vi "readLogStatusChecks.vi"(8 "error in (no error)":errorcluster, 10 "Parser":refnum<class "U8ArrayParserAutoIndexing.lvclass">, 11 "M1M3SAL in":refnum<class "M1M3SAL.lvclass">) -> (0 "error out":errorcluster, 2 "EventStatusChecks":variant, 3 "M1M3SAL out":refnum<class "M1M3SAL.lvclass">)   [LabVIEW 2016, in "M1M3SupportCommunicator.lvlib" / "M1M3SAL.lvclass"]
uses:
  M1M3SAL.lvclass
  Common_RT_Utilities/U8ArrayParserAutoIndexing/U8ArrayParserAutoIndexing.lvclass
  DataTypes/Topics/EventStatusChecks.ctl
  DataTypes/Topics/Parts/Timestamp.ctl
  DataTypes/Topics/M1M3SupportTopics.lvlib
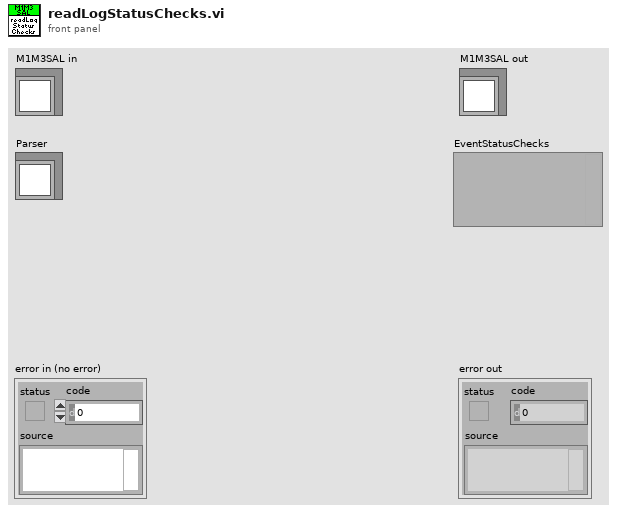
[diagram p1: front panel]
types:
  T1 = typedef "M1M3SupportTopics.lvlib/EventStatusChecks.ctl" = cluster{"Timestamp":T2, "ILCResetOk":bool, "DCAResetOk":bool, "ILCPowerOk":bool, "DCAPowerOk":bool}
  T2 = typedef "M1M3SupportTopics.lvlib/Timestamp.ctl" = dbl
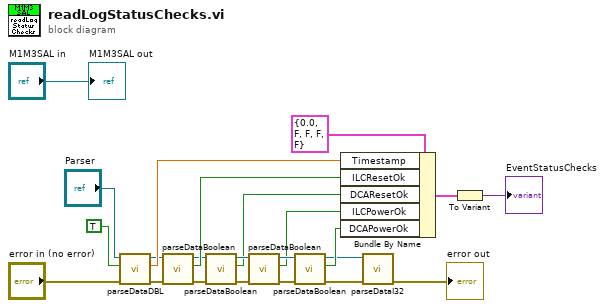
[diagram p0: block diagram]
diagram:
  n1 = call "parseDataDBL.vi"("error in (no error)"="error in (no error)", "OverrideSwapBytes"=TRUE, "U8ArrayParserAutoIndexing in"="Parser") -> ("error out"=w14:errorcluster, "Data"=w16:dbl, "U8ArrayParserAutoIndexing out"=w15:refnum<class "U8ArrayParserAutoIndexing.lvclass">)  [unwired: 6 in]
  n2 = call "parseDataBoolean.vi"("error in (no error)"=w14, "U8ArrayParserAutoIndexing in"=w15) -> ("error out"=w12:errorcluster, "Data"=w13:bool, "U8ArrayParserAutoIndexing out"=w11:refnum<class "U8ArrayParserAutoIndexing.lvclass">)  [unwired: 7 in]
  n3 = call "parseDataBoolean.vi"("error in (no error)"=w12, "U8ArrayParserAutoIndexing in"=w11) -> ("error out"=w10:errorcluster, "Data"=w6:bool, "U8ArrayParserAutoIndexing out"=w9:refnum<class "U8ArrayParserAutoIndexing.lvclass">)  [unwired: 7 in]
  n4 = call "parseDataBoolean.vi"("error in (no error)"=w10, "U8ArrayParserAutoIndexing in"=w9) -> ("error out"=w8:errorcluster, "Data"=w5:bool, "U8ArrayParserAutoIndexing out"=w7:refnum<class "U8ArrayParserAutoIndexing.lvclass">)  [unwired: 7 in]
  n5 = call "parseDataBoolean.vi"("error in (no error)"=w8, "U8ArrayParserAutoIndexing in"=w7) -> ("error out"=w1:errorcluster, "Data"=w4:bool, "U8ArrayParserAutoIndexing out"=w2:refnum<class "U8ArrayParserAutoIndexing.lvclass">)  [unwired: 7 in]
  n6 = Bundle By Name(cluster=T1 {"Timestamp"=0.0, "ILCResetOk"=FALSE, "DCAResetOk"=FALSE, "ILCPowerOk"=FALSE, "DCAPowerOk"=FALSE} ("EventStatusChecks"), "Timestamp"=w16, "ILCResetOk"=w13, "DCAResetOk"=w6, "ILCPowerOk"=w5, "DCAPowerOk"=w4) -> (w22:T1)
  n7 = call "parseDataI32.vi"("error in (no error)"=w1, "U8ArrayParserAutoIndexing in"=w2) -> ("error out"=→"error out":errorcluster)  [unwired: 7 in, 2 out]
  n8 = To Variant(anything=w22) -> (Variant=→"EventStatusChecks":variant)
  "M1M3SAL out" <- "M1M3SAL in"
